vi "Unlock.vi"(8 "error in (no error)":errorcluster, 11 "References":T1) -> (0 "error out":errorcluster, 3 "References Out":T1)   [LabVIEW 2019, in "Lock Library.lvlib"]
uses:
  Lock Library.lvlib
  References.ctl
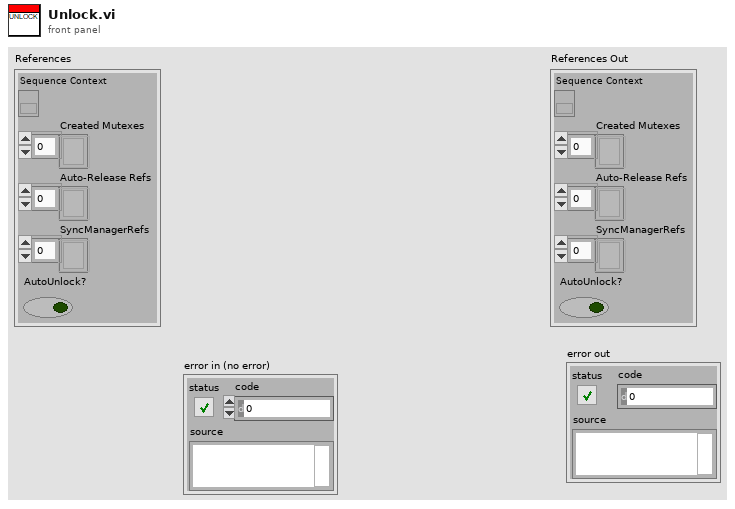
[diagram p1: front panel]
types:
  T1 = typedef "Lock Library.lvlib/References.ctl" = cluster{"Sequence Context":refnum<k7>, "Created Mutexes":refnum<k7>[], "Auto-Release Refs":refnum<k7>[], "SyncManagerRefs":refnum<k7>[], "AutoUnlock?":bool}
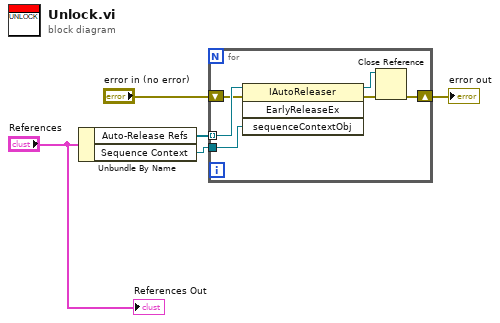
[diagram p0: block diagram]
diagram:
  n1 = Unbundle By Name("References") -> ("Auto-Release Refs"=w2:refnum<k7>[], "Sequence Context"=w1:refnum<k7>)
  n2 = for {
    tunnel: w2 -> [w11] mode=indexing
    tunnel: w1 -> [w10]
    shift-right: [w7] -> w5
    shift-left: "error in (no error)" -> [w8]
    n3 = invoke class="IAutoReleaser" method="EarlyReleaseEx"(reference=w11, error in=w8, "sequenceContextObj"=w10) -> (reference out=w6:refnum<k7>, error out=w9:errorcluster)  [unwired: 1 in, 2 out]
    n4 = Close Reference(reference=w6, error in (no error)=w9) -> (error out=w7:errorcluster)
  }
  "error out" <- w5
  "References Out" <- "References"
